vi "Single Freq Gen-4ch.vi"(7 "Stop Single Frquency":bool, 8 "error in (no error)":errorcluster, 10 "Amplitude":T1 {"Ch 4" max=255 step=1; "Ch 3" max=255 step=1; "Ch 2" max=255 step=1; "Ch 1" max=255 step=1}, 11 "Frequency (MHz)":T2 {"Ch 4" min=20 max=50 step=1; "Ch 3" min=20 max=50 step=1; "Ch 2" min=20 max=50 step=1; "Ch 1" min=20 max=50 step=1}) -> (0 "error out":errorcluster, 3 "Hex String (Array)":string[](array[string]))   [LabVIEW 2020]
uses:
  TypeDef/Frequency-4ch.ctl
  TypeDef/Amplitude-4ch.ctl
  Globals/FPGA Globals.vi
panel:
  out "Hex String 1":string
  out "Hex Length 1":i32
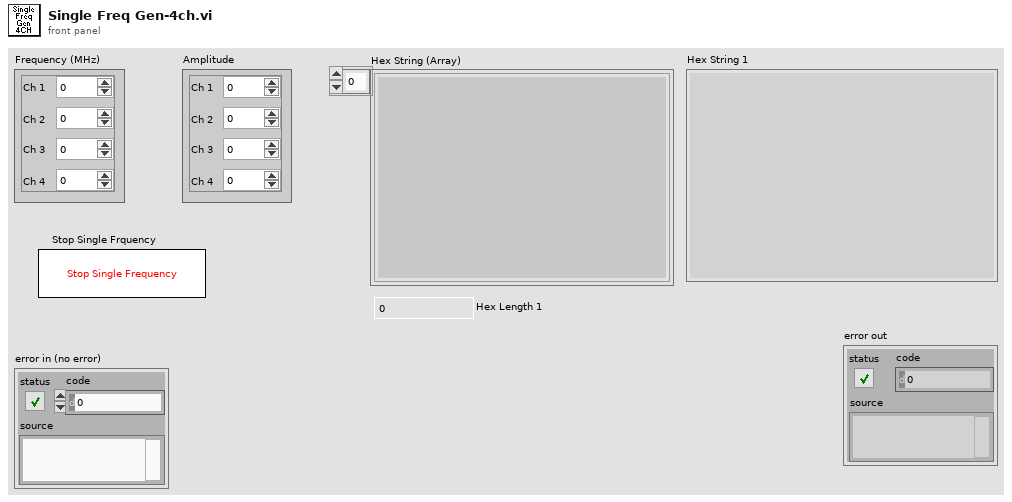
[diagram p1: front panel]
types:
  T1 = typedef "Amplitude-4ch.ctl" = cluster{"Ch 1":u16, "Ch 2":u16, "Ch 3":u16, "Ch 4":u16}
  T2 = typedef "Frequency-4ch.ctl" = cluster{"Ch 1":u16, "Ch 2":u16, "Ch 3":u16, "Ch 4":u16}
  T3 = typedef "FPGA Settings.ctl" = cluster{"System Clock(MHz)":dbl, "FPGA MAC 1":string, "Port Number 1":i32, "Port Number 2":i32, "FPGA MAC 2":string, "PC MAC Address":string}
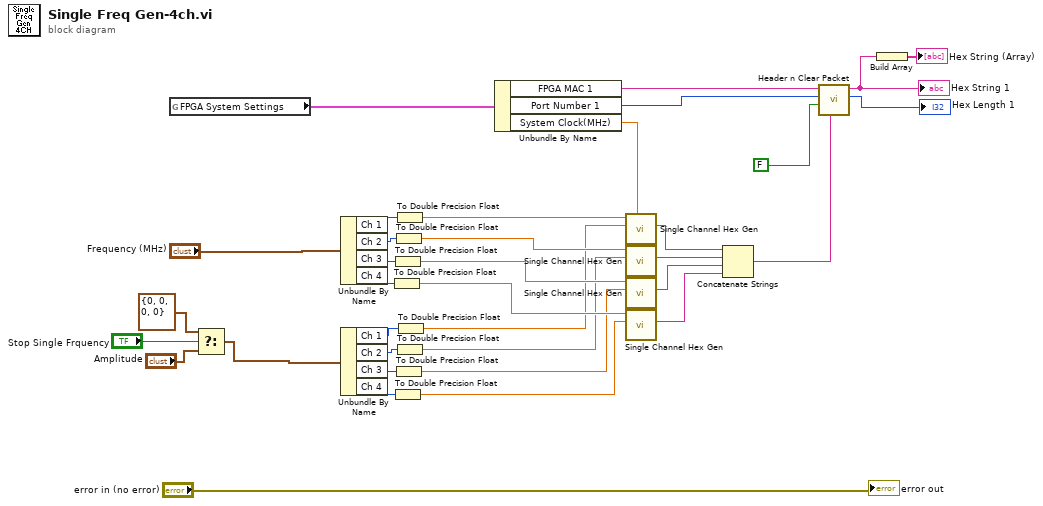
[diagram p0: block diagram]
diagram:
  n1 = global read "FPGA Globals.vi" "FPGA System Settings"() -> (w9:T3)
  n2 = Select(t=T1 {"Ch 1"=0, "Ch 2"=0, "Ch 3"=0, "Ch 4"=0} ("Amplitude 2"), s="Stop Single Frquency", f="Amplitude") -> (s? t:f=w5:T1)
  n3 = Unbundle By Name("Frequency (MHz)") -> ("Ch 1"=w31:u16, "Ch 2"=w29:u16, "Ch 3"=w27:u16, "Ch 4"=w25:u16)
  n4 = Unbundle By Name(w5) -> ("Ch 1"=w20:u16, "Ch 2"=w21:u16, "Ch 3"=w22:u16, "Ch 4"=w23:u16)
  n5 = To Double Precision Float(number=w25) -> (double precision float=w24:dbl)
  n6 = To Double Precision Float(number=w27) -> (double precision float=w26:dbl)
  n7 = To Double Precision Float(number=w23) -> (double precision float=w16:dbl)
  n8 = To Double Precision Float(number=w29) -> (double precision float=w28:dbl)
  n9 = To Double Precision Float(number=w22) -> (double precision float=w17:dbl)
  n10 = To Double Precision Float(number=w31) -> (double precision float=w30:dbl)
  n11 = To Double Precision Float(number=w21) -> (double precision float=w18:dbl)
  n12 = To Double Precision Float(number=w20) -> (double precision float=w19:dbl)
  n13 = Unbundle By Name(w9) -> ("FPGA MAC 1"=w12:string, "Port Number 1"=w11:i32, "System Clock(MHz)"=w10:dbl)
  n14 = call "Single Channel Hex Gen.vi"("System Clock(MHz)"=w10, "Amplitude"=w19, "Frequency"=w30) -> ("Single Freq Hex String"=w35:string)  [unwired: 8 in]
  n15 = call "Single Channel Hex Gen.vi"("System Clock(MHz)"=w10, "Amplitude"=w18, "Frequency"=w28) -> ("Single Freq Hex String"=w34:string)  [unwired: 8 in]
  n16 = call "Single Channel Hex Gen.vi"("System Clock(MHz)"=w10, "Amplitude"=w17, "Frequency"=w26) -> ("Single Freq Hex String"=w33:string)  [unwired: 8 in]
  n17 = call "Single Channel Hex Gen.vi"("System Clock(MHz)"=w10, "Amplitude"=w16, "Frequency"=w24) -> ("Single Freq Hex String"=w32:string)  [unwired: 8 in]
  n18 = Concatenate Strings(w35, w34, w33, w32) -> (w13:string)
  n19 = call "Header n Clear Packet.vi"("Hex String in"=w13, "Stop Single Frquency"=FALSE, "Port Number"=w11, "FPGA MAC"=w12) -> ("Hex Length"=→"Hex Length 1":i32, "Hex String out"=w3:string)  [unwired: 6 in]
  "Hex String 1" <- w3
  n20 = Build Array(w3) -> (→"Hex String (Array)":string[])
  "error out" <- "error in (no error)"
